vi "Strings to Cluster Ref.vi"(0 "control reference":refnum<vi>, 7 "Params":string[](array[string]), 11 "error in (no error)":errorcluster) -> (4 "control ref out":refnum<vi>, 15 "error out":errorcluster)   [LabVIEW 2020]
doc: "Parses a string to assign values to a cluster's controls."
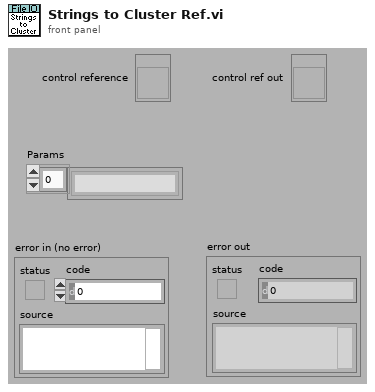
[diagram p1: front panel]
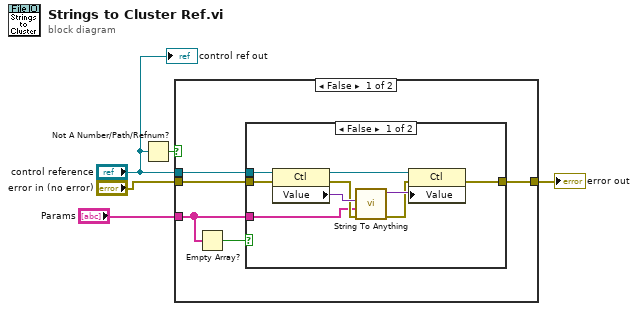
[diagram p0: block diagram]
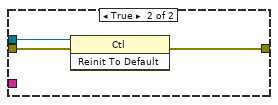
[diagram p2: hidden frame]
diagram:
  n1 = Not A Number/Path/Refnum?(number/path/refnum="control reference") -> (NaN/Path/Refnum?=w3:bool)
  n2 = case shown="False" w3 {
    tunnel: "Params" -> [w10 _]
    tunnel: [w6 w23] -> w5
    tunnel: "control reference" -> [w8 _]
    tunnel: "error in (no error)" -> [w7 w23]
    frame False {
      n3 = Empty Array?(array=w10) -> (empty?=w9:bool)
      n4 = case shown="False" w9 {
        tunnel: w10 -> [w11 _]
        tunnel: w8 -> [w19 w20]
        tunnel: w7 -> [w18 w22]
        tunnel: [w16 w21] -> w6
        frame False {
          n5 = property class="Ctl"(reference=w19, error in=w18) -> (reference out=w17:refnum<vi>, error out=w13:errorcluster, "Value"=w15:variant)
          n6 = call "String To Anything.vi"("Error In"=w13, "Strings"=w11, "Type of Anything"=w15) -> ("Error Out"=w12:errorcluster, "Variant"=w14:variant)  [unwired: 7 in]
          n7 = property class="Ctl"(reference=w17, error in=w12, "Value"=w14) -> (error out=w16:errorcluster)  [unwired: 1 out]
        }
        frame True {
          n8 = invoke class="Ctl" method="Reinit To Default"(reference=w20, error in=w22) -> (error out=w21:errorcluster)  [unwired: 1 in, 2 out]
        }
      }
    }
    frame True {
    }
  }
  "error out" <- w5
  "control ref out" <- "control reference"
